vi "senor input.vi"() -> ()   [LabVIEW 2012]
uses:
  <vilib>/robotics/Navigation/shared/WorldMap/OccupancyGridWorldMap/NI_Robotics_OccupancyGridWorldMap.lvclass
  <vilib>/rvi/interface/nirviReadWriteControl/nirviReadWriteControl.xnode
  NiFpgaLv.dll
  <vilib>/Utility/error.llb/Error Cluster From Error Code.vi
  <vilib>/rvi/interface/Simulation/niFpgaSimulationCallBeginRW.vi
  <vilib>/rvi/errors/niLvFpgaAdjustHostInterfaceError.vi
  <vilib>/rvi/interface/nirviOpenFPGA/nirviOpenFPGA.xnode
  <vilib>/rvi/interface/nirviCloseFPGA/nirviCloseFPGA.xnode
  <vilib>/FPGAPlugInAG/Dynamic/niLvFpga_Close_Dynamic.vi
  fpgatrig.vi
  <vilib>/rvi/interface/RandomDataEmulation/nirviRandomDataOpen.vi
  <vilib>/rvi/interface/common/niFpgaCacheSessionInfoDynamic.vi
panel:
  out "path on obstacles":dbl[][](graph)
  in  "stop":bool
  out "Rounded y":fxp<+/-,64,32>
  out "Rounded x":fxp<+/-,64,32>
  out "Detected x":fxp<+/-,64,32>
  out "Detected y":fxp<+/-,64,32>
  in  "Sensor x":fxp<+/-,64,32>
  in  "sensor y":fxp<+/-,64,32>
  in  "Radians":fxp<+/-,64,32>
  in  "distance":fxp<+/-,64,32>
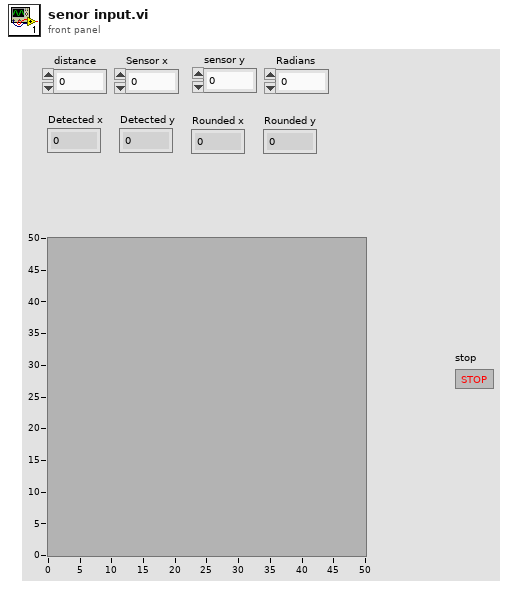
[diagram p1: front panel]
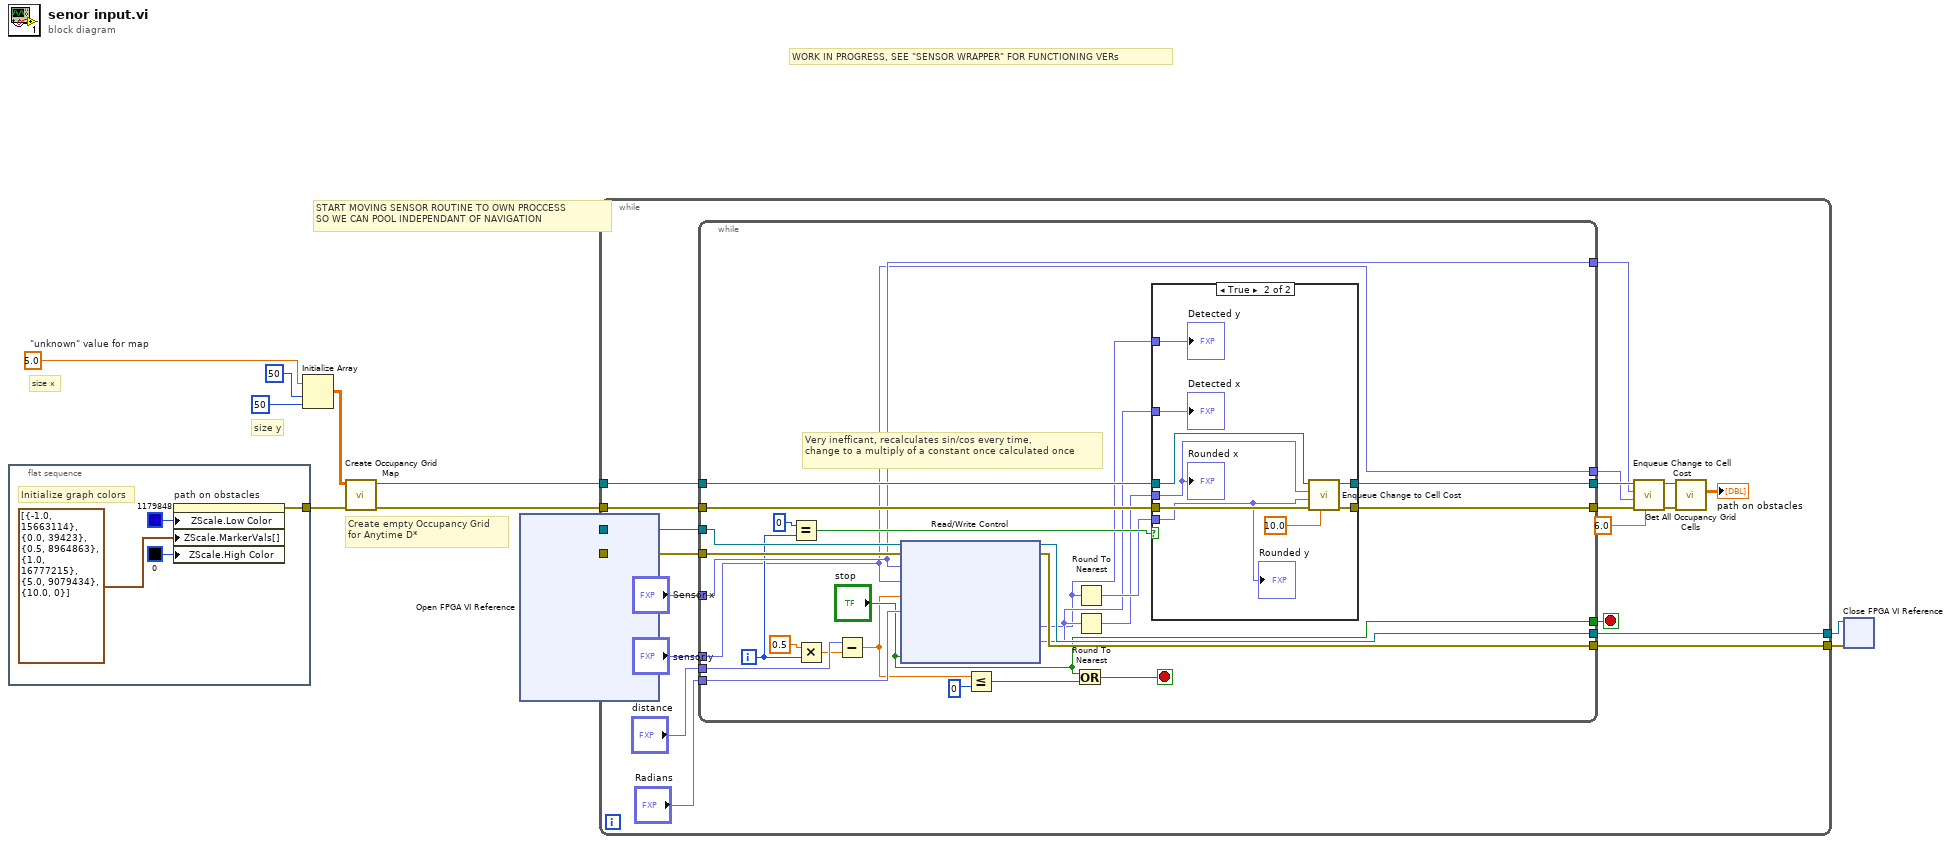
[diagram p0: block diagram]
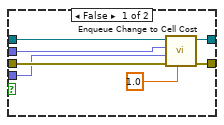
[diagram p2: hidden frame]
diagram:
  w5 = 5.0  # "unknown" value for map
  # "WORK IN PROGRESS, SEE \"SENSOR WRAPPER\" FOR FUNCTIONING VERs"
  # "START MOVING SENSOR ROUTINE TO OWN PROCCESS\nSO WE CAN POOL INDEPENDANT OF NAVIGATION"
  # "size y"
  # "size x"
  # "Create empty Occupancy Grid\nfor Anytime D*"
  n1 = flat-sequence {
    tunnel: [w12] -> w1
    frame #0 {
      # "Initialize graph colors"
      n2 = property on="path on obstacles" class="IntGraph (strict)"("ZScale.Low Color"=u32 1179848, "ZScale.MarkerVals[]"=cluster{dbl, u32}[] [{-1.0, 15663114}, {0.0, 39423}, {0.5, 8964863}, {1.0, 16777215}, {5.0, 9079434}, {10.0, 0}], "ZScale.High Color"=u32 0) -> (error out=w12:errorcluster)  [unwired: 2 in, 1 out]
    }
  }
  n3 = Initialize Array(w5, 50 ("y"), 50 ("x")) -> (w4:dbl[][])
  n4 = call <vilib>:"Create Occupancy Grid Map.vi"("error in (no error)"=w1, "occupancy grid"=w4) -> ("error out"=w2:errorcluster, "map reference out"=w3:refnum<data-value>)  [unwired: 8 in]
  n5 = xnode "Open FPGA VI Reference"() -> ("FPGA VI Reference Out"=w9:refnum<k20>, "error out"=w8:errorcluster)  [unwired: 2 in]
  n6 = while {
    tunnel: [w34] -> w11
    tunnel: w9 -> [w33]
    tunnel: w8 -> [w32]
    tunnel: [w31] -> w10
    tunnel: w3 -> [w29]
    tunnel: w2 -> [w28]
    stop <- w30 stop-if-true
    n7 = while {
      tunnel: [w60] -> w34
      tunnel: w33 -> [w59]
      tunnel: w32 -> [w58]
      tunnel: [w57] -> w31
      tunnel: ["stop"] -> w30
      tunnel: w29 -> [w56]
      tunnel: w28 -> [w55]
      tunnel: [w54] -> w26
      tunnel: [w53] -> w25
      tunnel: [w37] -> w24
      tunnel: [w50] -> w23
      tunnel: "sensor y" -> [w37]
      tunnel: "Sensor x" -> [w50]
      tunnel: "Radians" -> [w49]
      tunnel: "distance" -> [w41]
      i -> [w40]
      stop <- w43 stop-if-true
      # "Very inefficant, recalculates sin/cos every time, \nchange to a multiply of a constant once calculated once"
      n8 = Equal?(x=0, y=w40) -> (x = y?=w51:bool)
      n9 = Multiply(x=0.5, y=w40) -> (x*y=w38:dbl)
      n10 = Subtract(x=w41, y=w38) -> (x-y=w35:dbl)
      n11 = xnode "Read/Write Control"("FPGA VI Reference In"=w59, "error in"=w58, "Sensor position x"=w50, "Sensor position y"=w37, "Distance detected"=w35, "sensor angle (Radiens)"=w49, "stop"="stop") -> ("FPGA VI Reference Out"=w57:refnum<k20>, "error out"=w60:errorcluster, "Detected y Cord"=w45:fxp<+/-,64,32>, "Detected x Cord"=w46:fxp<+/-,64,32>)
      n12 = Less Or Equal?(x=w35, y=0) -> (x <= y?=w44:bool)
      n13 = Or(x="stop", y=w44) -> (x .or. y?=w43:bool)
      n14 = Round To Nearest(number=w45) -> (nearest integer value=w48:fxp<+/-,33,33>)
      n15 = Round To Nearest(number=w46) -> (nearest integer value=w47:fxp<+/-,33,33>)
      n16 = case shown="True" w51 {
        tunnel: w56 -> [w63 w76]
        tunnel: w55 -> [w64 w75]
        tunnel: [w66 w73] -> w54
        tunnel: [w65 w72] -> w53
        tunnel: w47 -> [w62 w68]
        tunnel: w48 -> [w61 w69]
        tunnel: w46 -> [_ w71]
        tunnel: w45 -> [_ w70]
        frame False {
          n17 = call <vilib>:"Enqueue Change to Cell Cost.vi"("cost"=1.0, "error in (no error)"=w64, "y"=w61, "x"=w62, "map reference in"=w63) -> ("error out"=w65:errorcluster, "map reference out"=w66:refnum<data-value>)  [unwired: 5 in]
        }
        frame True {
          n18 = call <vilib>:"Enqueue Change to Cell Cost.vi"("cost"=10.0, "error in (no error)"=w75, "y"=w69, "x"=w68, "map reference in"=w76) -> ("error out"=w72:errorcluster, "map reference out"=w73:refnum<data-value>)  [unwired: 5 in]
          "Rounded y" <- w69
          "Rounded x" <- w68
          "Detected x" <- w71
          "Detected y" <- w70
        }
      }
    }
    n19 = call <vilib>:"Enqueue Change to Cell Cost.vi"("cost"=6.0, "error in (no error)"=w25, "y"=w24, "x"=w23, "map reference in"=w26) -> ("error out"=w21:errorcluster, "map reference out"=w22:refnum<data-value>)  [unwired: 5 in]
    n20 = call <vilib>:"Get All Occupancy Grid Cells.vi"("error in (no error)"=w21, "map reference in"=w22) -> ("occupancy grid"=→"path on obstacles":dbl[][])  [unwired: 7 in, 2 out]
  }
  n21 = xnode "Close FPGA VI Reference"("FPGA VI Reference In"=w10, "error in"=w11) -> ()  [unwired: 1 out]
